vi "Measure vs B2Dv10.vi"() -> ()   [LabVIEW 2009]
doc: "This VI is an example operator panel.\n\nThe VI contains a table for the field values that may be configured manually, or loaded by checking the \"Prompt for File\" box. The data file should contain 3 columns of data, with each column delimited by a tab character.\n\nBefore the VI is executed, set the desired field units and coordinate system. Once the VI is started, follow the directions in the STATUS indicator to operate. Once a field value is achieved, it will be held indefinitely with no user intervention.\n\nThe present field is displayed in the selected units and coordinate system. The present field is queried once per second.\n\nIf a field point is specified that is outside the limits for the magnet, the VI will abort execution."
uses:
  <vilib>/Utility/file.llb/Read From Spreadsheet File (DBL).vi
panel:
  in  "AH":bool=TRUE
  in  "GPIB HP 2":string="13"
  in  "Wait between \nVectors":bool
  in  "Change\nPID\n(DetermineSIMPID.vi)":bool
  in  "Wait between \nVectors (ms)":u32=3000
  in  "X Axis":enum16{"B", "phi"}(ring)
  in  "Y Axis":T1(ring)=enum."HP (V)2"
  out "measured data":dbl[][](array[numeric])
  out "XY Graph":T2(graph)
  in  "Notes:":string="Datum: 16.01.12, Uhrzeit: 14:00, Sweep 0.15T/min,(measurevsB2Dv10.vi)), kapazitive Messung, leerer Sensor #1649_1, Referenzmessung, T=0.3K, Winkel 15° , optischer Probenstab, Gestell entfernt" caption="Notizen:"
  out "Messfile Refnum":refnum<file>
  in  "Measurement File":path=path "D:/UserData/Matthias/Messungen/#1649_leer/120116/120116_#1649_135deg_M1.txt"
  in  "Sample name:":string="#1649_1, leer"
  in  "HP 1":bool
  in  "GPIB HP":string="14"
  in  "HP 2":bool
  in  "LI 3":bool
  in  "GPIB L 3":string="8"
  in  "LI 2":bool
  in  "GPIB L 2":string="8"
  in  "LI 1":bool
  in  "GPIB L 1":string="8"
  out "Number of lines":i32=3
  in  "Operation":u16(ring)=1 items=["Stepwise", "Continous"]
  out "Ramp Rate along Vector (T/min)":dbl=0.2123426648592312 format="%.3f"
  out "Current Ramp Rate Z (T/min)":dbl=0.15014787650686168 format="%.3f"
  out "Current Ramp Rate Y (T/min)":dbl=0.15015 format="%.3f"
  in  "User defined Ramp Rate (T/min)":bool=TRUE
  in  "User defined Ramp Rate (T/min)":dbl=0.22 format="%.3f"
  in  "Z-Axis Communications Config":T3={"GPIB address"=22, "GPIB bus"=1, "connection ID"=refnum, "IP"="111.111.111.1", "Active Comm Interface"=0, "Serial Port"="", "Programmer Type"=0} {"Programmer Type" items=["Model 430", "Model 420"]; "Active Comm Interface" items=["TCP/IP (Model 430 Only)", "RS232", "IEEE488"]}
  in  "Max Ramp Rate - Y Axis (A/s)":dbl=0.055 format="%.3f"
  in  "Max Ramp Rate - Z Axis (A/s)":dbl=0.19 format="%.3f"
  in  "Magnitude Limit (kG)":dbl=45.1 format="%.3f"
  in  "Y-Axis Communications Config":T3={"GPIB address"=22, "GPIB bus"=1, "connection ID"=refnum, "IP"="111.111.111.2", "Active Comm Interface"=0, "Serial Port"="", "Programmer Type"=0} {"Programmer Type" items=["Model 430", "Model 420"]; "Active Comm Interface" items=["TCP/IP (Model 430 Only)", "RS232", "IEEE488"]}
  out "Cartesian Display (T)":T4={"Y-Axis Field (T)"=-1e-05, "Z-Axis Field (T)"=2.9999999999999997e-05} {"Z-Axis Field (T)" format="%.3f"; "Y-Axis Field (T)" format="%.3f"}
  in  "Starting index":i32=2
  in  "Normal color":u32(colorbox)=11711154
  in  "Highlight color":u32(colorbox)=16711680
  in  "Prompt for File?":bool
  out "Continue Execution?":bool=TRUE
  out "error out":T5
  in  "error in":T5
  out "STATUS":string="Zeroing vector."
  in  "Ramping Control":u16(ring)=4 items=["NEXT VECTOR", "RAMPING", "HOLDING", "PAUSE", "ZERO"]
  out "Cartesian Display (kG)":T6 {"Z-Axis Field (kG)" format="%.3f"; "Y-Axis Field (kG)" format="%.3f"}
  in  "Field Values":string[][](table)=[["4", "135"], ["-4", "135"], ["0", "0"]]
  out "Switch Heaters":bool=TRUE
  out "Polar Display (T)":T7={"q (degrees)"=315.0, "Field Magnitude (T)"=1.4142135623730951e-05} {"Field Magnitude (T)" format="%.3f"; "q (degrees)" format="%.3f"}
  out "Polar Display (kG)":T8 {"Field Magnitude (kG)" format="%.3f"; "q (degrees)" format="%.3f"}
  in  "Coordinate System":u16(ring)=1 items=["Cartesian", "Polar"]
  in  "Magnetic Field Units":u16(ring)=1 items=["kG", "Tesla"]
  # "kontinuirliche Messung mit PID off bei 0, geht nur im Cartesian mode!"
  # "Measurement Display"
  # "Measurement Settings"
  # "Magnet Settings"
  # "Max Ramp Rate z: 1.27 T/min\nMax Ramp Rate y: 0.17 T/min"
  # "Devices"
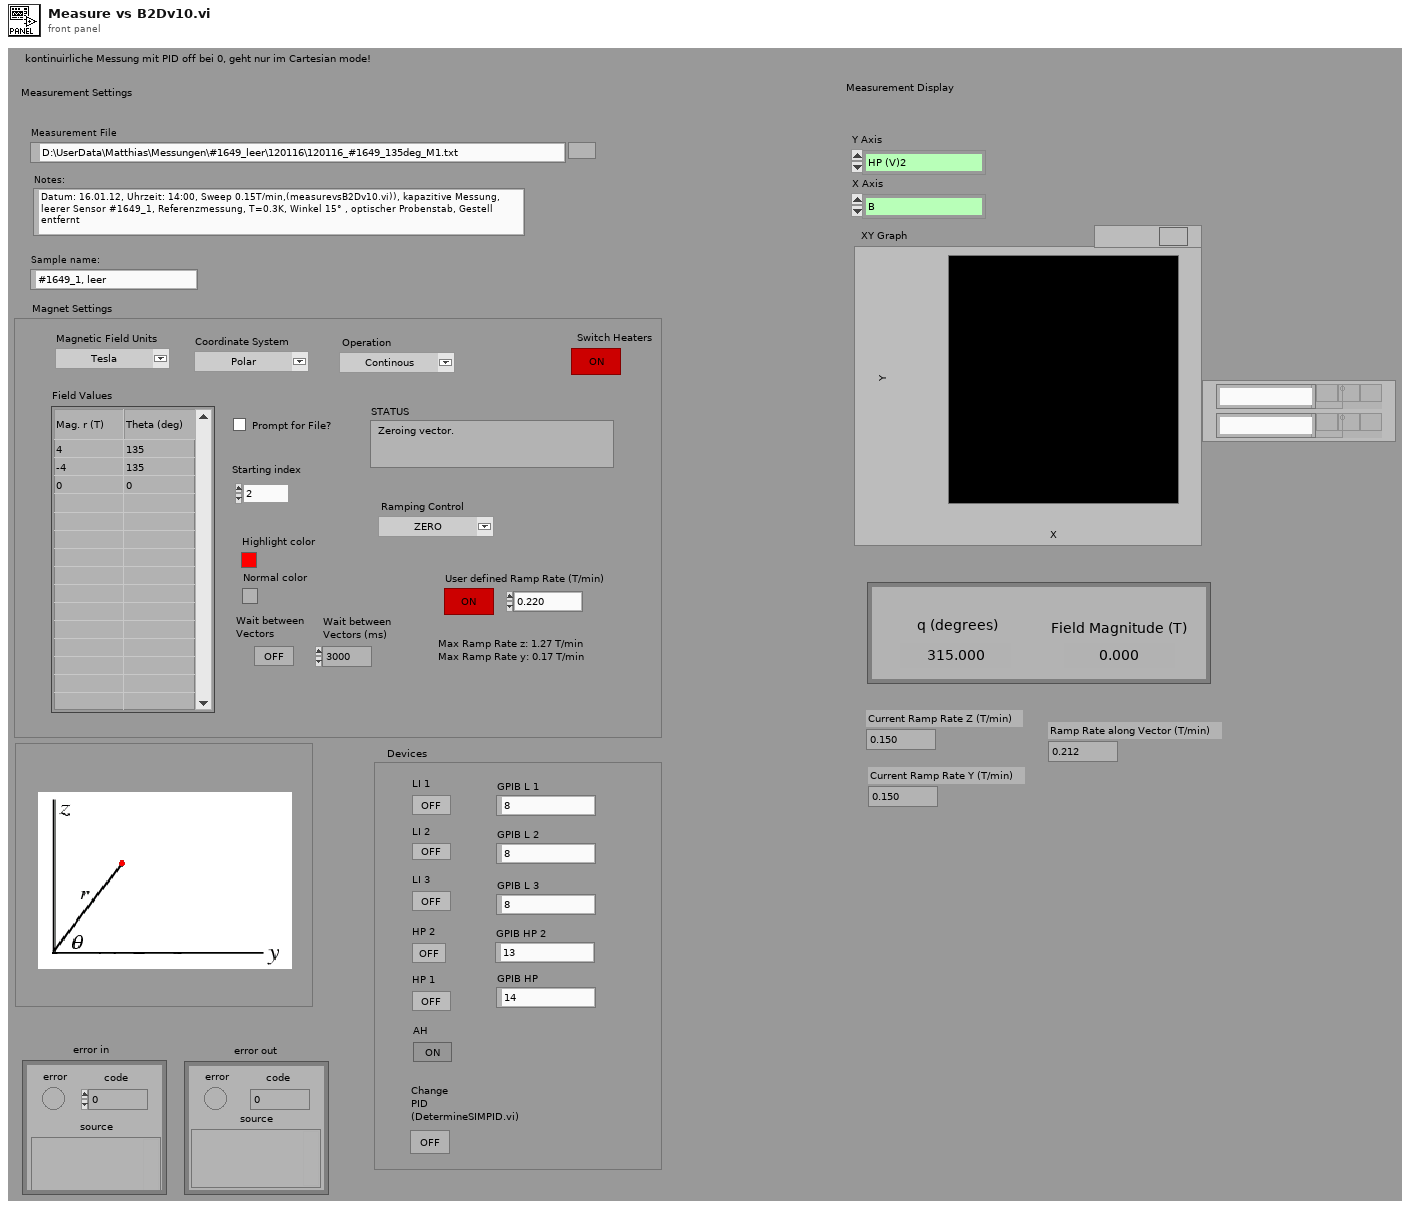
[diagram p1: front panel]
types:
  T1 = enum16{"B", "phi", "LI 1 Vx", "LI 1 phase", "LI 2 Vx", "LI 2 phase", "LI 3 Vx", "LI 3 phase", "LI 4 Vx", "LI 4 phase", "HP (V)", "HP (V)2", "AH C (pF)", "AH loss"}
  T2 = cluster{"measured data":dbl[], "measured data":dbl[]}
  T3 = cluster{"GPIB address":i16, "GPIB bus":i16, "connection ID":refnum<k5>, "IP":string, "Active Comm Interface":u16, "Serial Port":refnum<visa-resource-name>, "Programmer Type":u16}
  T4 = cluster{"Y-Axis Field (T)":dbl, "Z-Axis Field (T)":dbl}
  T5 = cluster{"error":bool, "code":i32, "source":string}
  T6 = cluster{"Y-Axis Field (kG)":dbl, "Z-Axis Field (kG)":dbl}
  T7 = cluster{"q (degrees)":dbl, "Field Magnitude (T)":dbl}
  T8 = cluster{"q (degrees)":dbl, "Field Magnitude (kG)":dbl}
  T9 = enum16{"", "RAMPING", "HOLDING", "PAUSED", "MANUAL UP", "MANUAL DOWN", "ZEROING CURRENT", "QUENCH DETECTED", "HEATING SWITCH"}
  T10 = enum16{"", "RAMPING", "HOLDING", "PAUSED", "MANUAL UP", "MANUAL DOWN", "ZEROING CURRENT", "QUENCH DETECTED", "HEATING SWITCH", "AT ZER0", "COOLING SWITCH"}
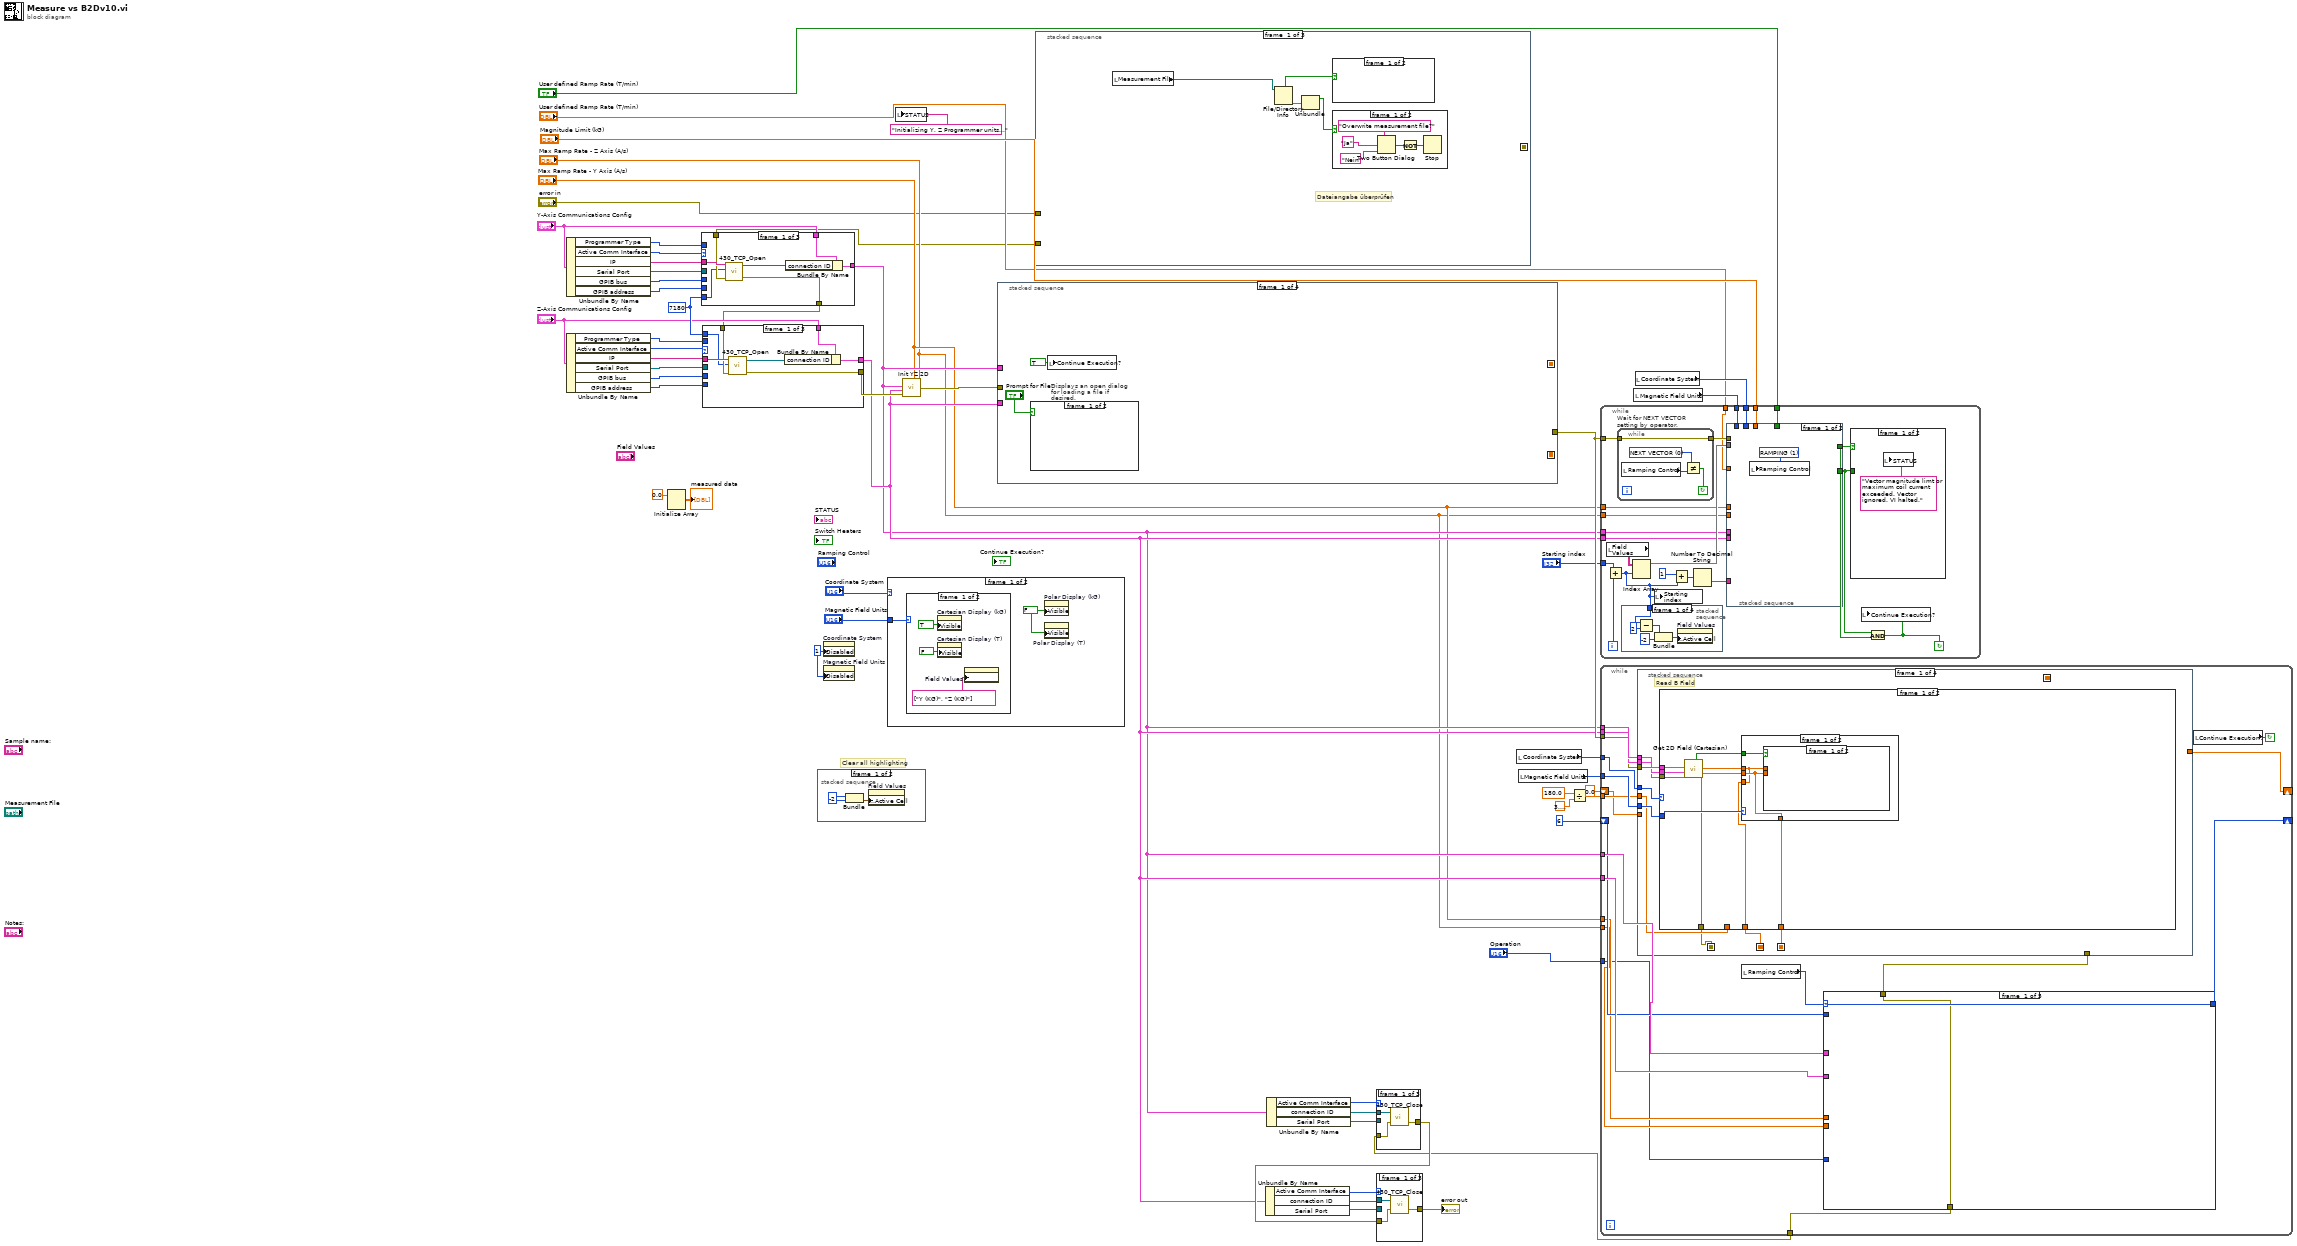
[diagram p0: block diagram]
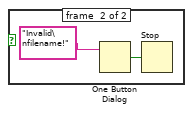
[diagram p3: hidden frame]
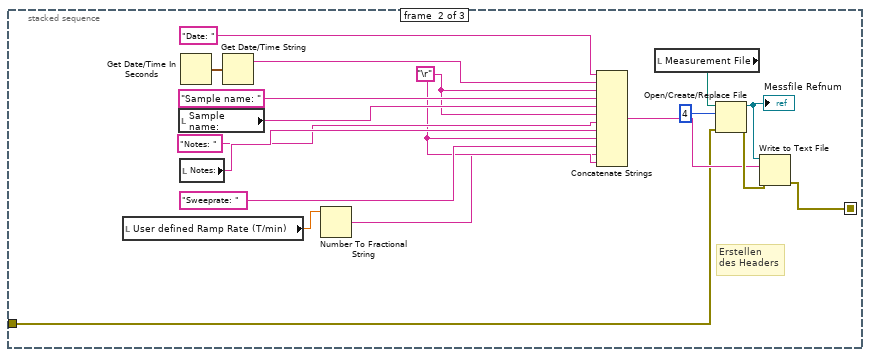
[diagram p4: hidden frame]
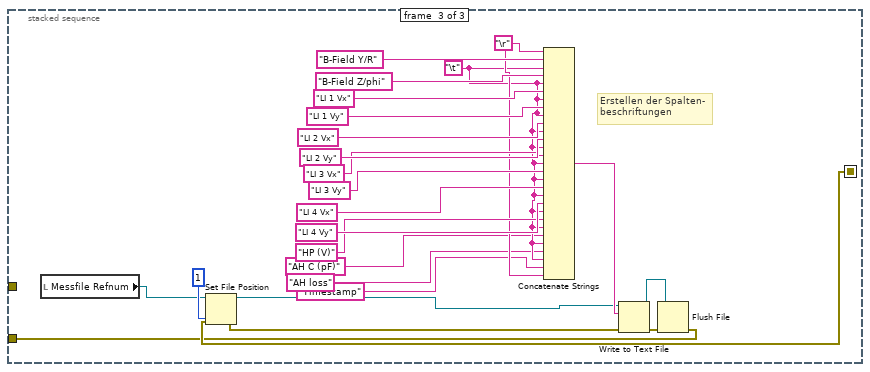
[diagram p5: hidden frame]
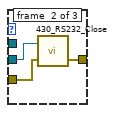
[diagram p6: hidden frame]
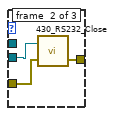
[diagram p8: hidden frame]
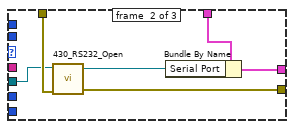
[diagram p10: hidden frame]
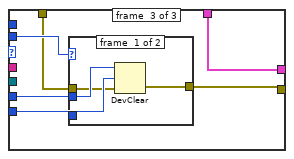
[diagram p11: hidden frame]
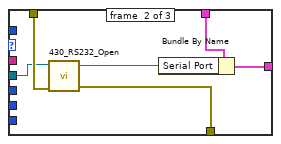
[diagram p13: hidden frame]
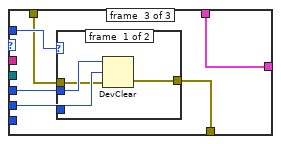
[diagram p14: hidden frame]
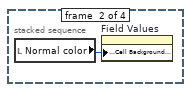
[diagram p16: hidden frame]
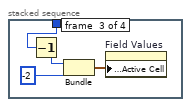
[diagram p17: hidden frame]
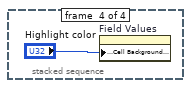
[diagram p18: hidden frame]
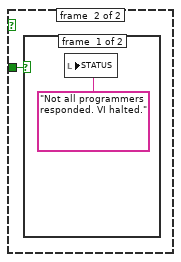
[diagram p19: hidden frame]
diagram:
  w39 = 7180 ("TCP Port")
  w52 = u8 1 ("Write Attribute")
  # "Clear all highlighting"
  n1 = Unbundle By Name("Z-Axis Communications Config") -> ("Programmer Type"=w15:u16, "Active Comm Interface"=w38:u16, "IP"=w35:string, "Serial Port"=w34:refnum<visa-resource-name>, "GPIB bus"=w14:i16, "GPIB address"=w13:i16)
  n2 = Unbundle By Name("Y-Axis Communications Config") -> ("Programmer Type"=w9:u16, "Active Comm Interface"=w37:u16, "IP"=w36:string, "Serial Port"=w33:refnum<visa-resource-name>, "GPIB bus"=w10:i16, "GPIB address"=w11:i16)
  n3 = Initialize Array(0.0 ("element")) -> (→"measured data":dbl[][])  [unwired: 2 in]
  n4 = stacked-sequence {
    frame #0 {
      w55 = -2
      n5 = Bundle(w55, w55) -> (w56:cluster{i32, i32})  [unwired: 1 in]
      n6 = property on="Field Values" class="Tbl (strict)"("Active Cell:Active Cell"=w56) -> ()  [unwired: 2 in, 2 out]
    }
    frame #1 {
      n7 = property on="Field Values" class="Tbl (strict)"("Active Cell:Cell Background Color"="Normal color") -> ()  [unwired: 2 in, 2 out]
    }
  }
  n8 = property on="Coordinate System" class="Ring (strict)"("Disabled"=w52) -> ()  [unwired: 2 in, 2 out]
  n9 = property on="Magnetic Field Units" class="Ring (strict)"("Disabled"=w52) -> ()  [unwired: 2 in, 2 out]
  n10 = case shown="0, Default" "Coordinate System" {
    tunnel: "Magnetic Field Units" -> [w59 w67]
    frame #0 {
      w58 = FALSE ("Write Attribute")
      (unwired) FALSE ("Write Attribute")
      (unwired) TRUE ("Write Attribute")
      n11 = case shown="1" w59 {
        frame #0 {
          n12 = property on="Cartesian Display (kG)" class="Cluster (strict)"("Visible"=TRUE ("Write Attribute")) -> ()  [unwired: 2 in, 2 out]
          n13 = property on="Cartesian Display (T)" class="Cluster (strict)"("Visible"=FALSE ("Write Attribute")) -> ()  [unwired: 2 in, 2 out]
          n14 = property on="Field Values" class="Tbl (strict)"("Column Header Strings[]"=string[] ["Y (KG)", "Z (KG)"] ("Write Attribute")) -> ()  [unwired: 2 in, 2 out]
        }
        frame #1 {
          n15 = property on="Cartesian Display (kG)" class="Cluster (strict)"("Visible"=FALSE ("Write Attribute")) -> ()  [unwired: 2 in, 2 out]
          n16 = property on="Cartesian Display (T)" class="Cluster (strict)"("Visible"=TRUE ("Write Attribute")) -> ()  [unwired: 2 in, 2 out]
          n17 = property on="Field Values" class="Tbl (strict)"("Column Header Strings[]"=string[] ["Y (T)", "Z (T)"] ("Write Attribute")) -> ()  [unwired: 2 in, 2 out]
        }
      }
      n18 = property on="Polar Display (kG)" class="Clust (strict)"("Visible"=w58) -> ()  [unwired: 2 in, 2 out]
      n19 = property on="Polar Display (T)" class="Clust (strict)"("Visible"=w58) -> ()  [unwired: 2 in, 2 out]
    }
    frame #1 {
      (unwired) FALSE ("Write Attribute")
      (unwired) TRUE ("Write Attribute")
      w66 = FALSE ("Write Attribute")
      n20 = case shown="1" w67 {
        frame #0 {
          n21 = property on="Polar Display (kG)" class="Clust (strict)"("Visible"=TRUE ("Write Attribute")) -> ()  [unwired: 2 in, 2 out]
          n22 = property on="Polar Display (T)" class="Clust (strict)"("Visible"=FALSE ("Write Attribute")) -> ()  [unwired: 2 in, 2 out]
          n23 = property on="Field Values" class="Tbl (strict)"("Column Header Strings[]"=string[] ["Mag. r (KG)", "Theta (deg)"] ("Write Attribute")) -> ()  [unwired: 2 in, 2 out]
        }
        frame #1 {
          n24 = property on="Polar Display (kG)" class="Clust (strict)"("Visible"=FALSE ("Write Attribute")) -> ()  [unwired: 2 in, 2 out]
          n25 = property on="Polar Display (T)" class="Clust (strict)"("Visible"=TRUE ("Write Attribute")) -> ()  [unwired: 2 in, 2 out]
          n26 = property on="Field Values" class="Tbl (strict)"("Column Header Strings[]"=string[] ["Mag. r (T)", "Theta (deg)"] ("Write Attribute")) -> ()  [unwired: 2 in, 2 out]
        }
      }
      n27 = property on="Cartesian Display (kG)" class="Cluster (strict)"("Visible"=w66) -> ()  [unwired: 2 in, 2 out]
      n28 = property on="Cartesian Display (T)" class="Cluster (strict)"("Visible"=w66) -> ()  [unwired: 2 in, 2 out]
    }
  }
  n29 = local write "STATUS"("Initializing Y, Z Programmer units..." ("STATUS")) -> ()
  n30 = stacked-sequence {
    seq-local: [_ w85 _] -> [_ _ w109]
    tunnel: "error in" -> [_ w86 _]
    tunnel: [_ _ w108] -> w4
    frame #0 {
      # "Dateiangabe überprüfen"
      n31 = local read "Measurement File"() -> (w77:path)
      n32 = File/Directory Info(path=w77) -> (directory=w75:bool, error out=w76:errorcluster)  [unwired: 1 in, 5 out]
      n33 = Unbundle(w76) -> ("status"=w74:bool)  [unwired: 2 out]
      n34 = case shown="False" w75 {
        frame #0 {
        }
        frame #1 {
          n35 = One Button Dialog(message="Invalid\nfilename!") -> (true=w83:bool)  [unwired: 1 in]
          n36 = Stop(stop? (T)=w83) -> ()
        }
      }
      n37 = case shown="False" w74 {
        frame #0 {
          n38 = Two Button Dialog(message="Overwrite measurement file?", 1:"Nein", 2:"Ja") -> (T button?=w79:bool)
          n39 = Not(x=w79) -> (.not. x?=w78:bool)
          n40 = Stop(stop? (T)=w78) -> ()
        }
        frame #1 {
        }
      }
    }
    frame #1 {
      w89 = "\r"
      # "Erstellen\ndes Headers"
      n41 = local read "User defined Ramp Rate (T/min)"() -> (w88:dbl)
      n42 = local read "Sample name:"() -> (w95:string)
      n43 = local read "Notes:"() -> (w97:string)
      n44 = Get Date/Time In Seconds() -> (seconds since 1Jan1904=w91:timestamp)
      n45 = Get Date/Time String(seconds (now)=w91) -> (date string=w93:string)  [unwired: 2 in, 1 out]
      n46 = Number To Fractional String(number=w88) -> (F-format string=w87:string)  [unwired: 3 in]
      n47 = Concatenate Strings("Date: ", w93, w89, "Sample name: ", w95, w89, "Notes: ", w97, w89, "Sweeprate: ", w87, w89) -> (w101:string)
      n48 = local read "Measurement File"() -> (w98:path)
      n49 = Open/Create/Replace File(file path (use dialog)=w98, error in=w86, operation (0:open)=4) -> (refnum out=w100:refnum<file>, error out=w102:errorcluster)  [unwired: 3 in, 1 out]
      "Messfile Refnum" <- w100
      n50 = Write to Text File(file (use dialog)=w100, text=w101, error in=w102) -> (error out=w85:errorcluster)  [unwired: 1 in, 2 out]
    }
    frame #2 {
      w105 = "\t"
      w107 = "\r"
      # "Erstellen der Spalten-\nbeschriftungen"
      n51 = local read "Messfile Refnum"() -> (w116:refnum<file>)
      n52 = Set File Position(refnum=w116, from (0:start)=1, error in=w109) -> (refnum out=w122:refnum<file>, error out=w124:errorcluster)  [unwired: 1 in]
      n53 = Concatenate Strings(w107, "B-Field Y/R", w105, "B-Field Z/phi", w105, "LI 1 Vx", w105, "LI 1 Vy", w105, "LI 2 Vx", w105, "LI 2 Vy", w105, "LI 3 Vx", w105, "LI 3 Vy", w105, "LI 4 Vx", w105, "LI 4 Vy", w105, "HP (V)", w105, "AH C (pF)" ("string"), w105, "AH loss" ("string"), w105, "Timestamp", w107) -> (w123:string)
      n54 = Write to Text File(file (use dialog)=w122, text=w123, error in=w124) -> (refnum out=w126:refnum<file>, error out=w125:errorcluster)  [unwired: 1 in, 1 out]
      n55 = Flush File(refnum=w126, error in=w125) -> (error out=w108:errorcluster)  [unwired: 1 out]
    }
  }
  n56 = case shown="0, Default" w37 {
    tunnel: w36 -> [w134 _ _]
    tunnel: w4 -> [w133 w140 w142]
    tunnel: "Y-Axis Communications Config" -> [w132 w135 w146]
    tunnel: [w130 w138 w146] -> w22
    tunnel: [w129 w139 w141] -> w12
    tunnel: w39 -> [w128 _ _]
    tunnel: w33 -> [_ w136 _]
    tunnel: w11 -> [_ _ w145]
    tunnel: w10 -> [_ _ w144]
    tunnel: w9 -> [_ _ w143]
    frame #0 {
      n57 = call <userlib>:"430_TCP_Open.vi"("IP Address"=w134, "TCP Port"=w128, "error in (no error)"=w133) -> ("connection ID"=w131:refnum<k5>, "error out"=w129:errorcluster)  [unwired: 3 in, 1 out]
      n58 = Bundle By Name(cluster=w132, "connection ID"=w131) -> (w130:T3)
    }
    frame #1 {
      n59 = call <userlib>:"430_RS232_Open.vi"("VISA resource name"=w136, "error in (no error)"=w140) -> ("VISA resource name out"=w137:refnum<visa-resource-name>, "error out"=w139:errorcluster)  [unwired: 5 in]
      n60 = Bundle By Name(cluster=w135, "Serial Port"=w137) -> (w138:T3)
    }
    frame #2 {
      n61 = case shown="1" w143 {
        tunnel: w144 -> [w150 _]
        tunnel: w145 -> [w149 _]
        tunnel: w142 -> [w148 w151]
        tunnel: [w147 w151] -> w141
        frame #0 {
          n62 = DevClear(2:w148, 3:w149, 4:w150) -> (0:w147:errorcluster)  [unwired: 1 out]
        }
        frame #1 {
        }
      }
    }
  }
  n63 = case shown="0, Default" w38 {
    tunnel: w35 -> [w158 _ _]
    tunnel: w12 -> [w157 w164 w166]
    tunnel: [w156 w163 w165] -> w32
    tunnel: "Z-Axis Communications Config" -> [w155 w161 w170]
    tunnel: [w153 w162 w170] -> w23
    tunnel: w39 -> [w152 _ _]
    tunnel: w34 -> [_ w159 _]
    tunnel: w15 -> [_ _ w169]
    tunnel: w14 -> [_ _ w168]
    tunnel: w13 -> [_ _ w167]
    frame #0 {
      n64 = call <userlib>:"430_TCP_Open.vi"("IP Address"=w158, "TCP Port"=w152, "error in (no error)"=w157) -> ("connection ID"=w154:refnum<k5>, "error out"=w156:errorcluster)  [unwired: 3 in, 1 out]
      n65 = Bundle By Name(cluster=w155, "connection ID"=w154) -> (w153:T3)
    }
    frame #1 {
      n66 = call <userlib>:"430_RS232_Open.vi"("VISA resource name"=w159, "error in (no error)"=w164) -> ("VISA resource name out"=w160:refnum<visa-resource-name>, "error out"=w163:errorcluster)  [unwired: 5 in]
      n67 = Bundle By Name(cluster=w161, "Serial Port"=w160) -> (w162:T3)
    }
    frame #2 {
      n68 = case shown="0, Default" w169 {
        tunnel: w168 -> [w174 _]
        tunnel: w167 -> [w173 _]
        tunnel: w166 -> [w172 w175]
        tunnel: [w171 w175] -> w165
        frame #0 {
          n69 = DevClear(2:w172, 3:w173, 4:w174) -> (0:w171:errorcluster)  [unwired: 1 out]
        }
        frame #1 {
        }
      }
    }
  }
  n70 = call <userlib>:"Init YZ 2D.vi"("Max Ramp Rate Z-axis"="Max Ramp Rate - Z Axis (A/s)", "Max Ramp Rate Y-axis"="Max Ramp Rate - Y Axis (A/s)", "error in"=w32, "Z-Axis Communications Config"=w23, "Y-Axis Communications Config"=w22) -> ("error out"=w50:T5)  [unwired: 5 in]
  n71 = stacked-sequence {
    seq-local: [_ w183 _ _] -> [_ _ w230 _]
    seq-local: [_ w182 _ _] -> [_ _ w229 _]
    tunnel: w23 -> [_ w185 _ _]
    tunnel: w50 -> [_ w186 _ _]
    tunnel: [_ w181 _ _] -> w46
    tunnel: w22 -> [_ w184 _ _]
    frame #0 {
      n72 = case "Displays an open dialog for loading a file if desired." shown="True" "Prompt for File?" {
        frame #0 {
        }
        frame #1 {
          n73 = call-poly <vilib>:"Read From Spreadsheet File.vi"() -> ("all rows"=w180:dbl[][])  [unwired: 7 in, 4 out]
          n74 = Number To Fractional String(number=w180, precision (6)=i16 4) -> (F-format string=w179:string[][])  [unwired: 2 in]
          n75 = local write "Field Values"(w179) -> ()
        }
      }
      n76 = local write "Continue Execution?"(TRUE ("Continue Execution?")) -> ()
    }
    frame #1 {
      w194 = u16 3 items=["NEXT VECTOR", "RAMPING", "HOLDING", "PAUSE", "ZERO"] ("Ramping Control")
      n77 = call <userlib>:"Get Switch Present.vi"("error in"=w186, "Communications Config"=w184) -> ("error out"=w190:T5, "Switch Present?"=w191:bool)
      n78 = case shown="True" w191 {
        tunnel: w190 -> [w212 w221]
        tunnel: w184 -> [_ w214]
        tunnel: [0.0 w218] -> w182
        tunnel: [w212 w220] -> w189
        frame #0 {
        }
        frame #1 {
          n79 = call <userlib>:"Get Switch Heater Time.vi"("error in"=w221, "Communications Config"=w214) -> ("error out"=w217:T5, "Switch Heating Time (secs)"=w219:dbl)
          n80 = call <userlib>:"Get Switch Heater.vi"("error in"=w217, "Communications Config"=w214) -> ("error out"=w216:T5, "Switch Heater Indicator"=w215:bool)
          n81 = case shown="False" w215 {
            tunnel: [w226 w227] -> w220
            tunnel: w219 -> [w224 _]
            tunnel: [w224 0.0] -> w218
            tunnel: w216 -> [w222 w227]
            tunnel: w214 -> [w223 _]
            frame #0 {
              n82 = call <userlib>:"Set Switch Heater.vi"("error in"=w222, "Switch Heater Control"=TRUE, "Communications Config"=w223) -> ("error out"=w226:T5)
            }
            frame #1 {
            }
          }
        }
      }
      n83 = call <userlib>:"Get Switch Present.vi"("error in"=w189, "Communications Config"=w185) -> ("error out"=w187:T5, "Switch Present?"=w188:bool)
      n84 = case shown="True" w188 {
        tunnel: w187 -> [w195 w204]
        tunnel: w185 -> [_ w197]
        tunnel: [0.0 w201] -> w183
        tunnel: [w195 w203] -> w181
        frame #0 {
        }
        frame #1 {
          n85 = call <userlib>:"Get Switch Heater Time.vi"("error in"=w204, "Communications Config"=w197) -> ("error out"=w200:T5, "Switch Heating Time (secs)"=w202:dbl)
          n86 = call <userlib>:"Get Switch Heater.vi"("error in"=w200, "Communications Config"=w197) -> ("error out"=w199:T5, "Switch Heater Indicator"=w198:bool)
          n87 = case shown="False" w198 {
            tunnel: [w205 w210] -> w203
            tunnel: w202 -> [w208 _]
            tunnel: [w208 0.0] -> w201
            tunnel: w199 -> [w206 w210]
            tunnel: w197 -> [w207 _]
            frame #0 {
              n88 = call <userlib>:"Set Switch Heater.vi"("error in"=w206, "Switch Heater Control"=TRUE, "Communications Config"=w207) -> ("error out"=w205:T5)
            }
            frame #1 {
            }
          }
        }
      }
      n89 = local write "Ramping Control"(w194) -> ()
      n90 = local write "Switch Heaters"(TRUE ("Switch Heater Control")) -> ()
      n91 = property on="Switch Heaters" class="Boolean (strict)"("Disabled"=u8 1 ("Write Attribute")) -> ()  [unwired: 2 in, 2 out]
    }
    frame #2 {
      n92 = Max & Min(x=w230, y=w229) -> (max(x,y)=w231:dbl)  [unwired: 1 out]
      n93 = local write "STATUS"("Heating switches..." ("STATUS")) -> ()
      n94 = Add(x=w231, y=2) -> (x+y=w235:dbl)
      n95 = property on="Ramping Control" class="Ring (strict)"("Disabled"=u8 1 ("Write Attribute")) -> ()  [unwired: 2 in, 2 out]
      n96 = Multiply(x=w235, y=1000) -> (x*y=w234:dbl)
      n97 = Wait (ms)(milliseconds to wait=w234) -> ()  [unwired: 1 out]
    }
    frame #3 {
      n98 = property on="Ramping Control" class="Ring (strict)"("Disabled"=u8 0 ("Write Attribute")) -> ()  [unwired: 2 in, 2 out]
      n99 = local write "STATUS"("Ready to ramp to first vector. Set Ramping Mode to NEXT VECTOR to begin." ("STATUS")) -> ()
      n100 = local read "Field Values"() -> (w240:string[][])
      n101 = Array Size(array=w240) -> (size(s)=w239:i32[])
      n102 = Index Array(array=w239, index=0) -> (element=→"Number of lines":i32)
    }
  }
  n103 = Unbundle By Name(w23) -> ("Active Comm Interface"=w29:u16, "connection ID"=w28:refnum<k5>, "Serial Port"=w27:refnum<visa-resource-name>)
  n104 = Unbundle By Name(w22) -> ("Active Comm Interface"=w30:u16, "connection ID"=w26:refnum<k5>, "Serial Port"=w25:refnum<visa-resource-name>)
  n105 = local read "Coordinate System"() -> (w47:u16)
  n106 = local read "Magnetic Field Units"() -> (w45:u16)
  n107 = Divide(x=180.0, y=3.141592653589793) -> (x/y=w42:dbl)
  n108 = while {
    shift-left: u16 6 ("Ramping Control") -> [w250]
    shift-right: [w251] -> _
    tunnel: [w253] -> w24
    tunnel: w23 -> [w254]
    tunnel: w22 -> [w255]
    tunnel: w42 -> [w257]
    tunnel: w45 -> [w258]
    tunnel: w46 -> [w259]
    tunnel: w23 -> [w260]
    tunnel: w22 -> [w261]
    tunnel: w47 -> [w262]
    tunnel: "Max Ramp Rate - Y Axis (A/s)" -> [w249]
    tunnel: "Max Ramp Rate - Z Axis (A/s)" -> [w248]
    tunnel: "Operation" -> [w247]
    shift-right: [w245] -> _
    shift-left: 0.0 -> [w244]
    stop <- w252 continue-if-true
    n109 = stacked-sequence {
      seq-local: [w265 _ _ _] -> [_ _ w389 _]
      seq-local: [w264 _ _ _] -> [_ w338 w386 _]
      seq-local: [w263 _ _ _] -> [_ w339 w387 _]
      seq-local: [_ _ w374 _] -> [_ _ _ w459]
      tunnel: w262 -> [w271 _ _ w457]
      tunnel: w261 -> [w270 _ _ _]
      tunnel: w260 -> [w269 _ _ _]
      tunnel: w259 -> [w268 _ _ _]
      tunnel: w258 -> [w267 _ _ _]
      tunnel: w257 -> [w266 _ _ _]
      tunnel: [_ _ w388 _] -> w246
      tunnel: [_ w341 _ _] -> w245
      tunnel: w244 -> [_ w340 _ _]
      frame #0 {
        # "Read B Field"
        n110 = case shown="0, Default" w271 {
          tunnel: w270 -> [w281 w304]
          tunnel: w269 -> [w280 w303]
          tunnel: w268 -> [w279 w302]
          tunnel: w267 -> [w278 w301]
          tunnel: w266 -> [_ w300]
          tunnel: [w274 w299] -> w265
          tunnel: [w273 w297] -> w264
          tunnel: [w272 w298] -> w263
          frame #0 {
            n111 = call <userlib>:"Get 2D Field (Cartesian).vi"("Y-Axis Communications Config"=w281, "Z-Axis Communications Config"=w280, "error in"=w279) -> ("All Instruments Responded?"=w275:bool, "Y-Axis Field (kG)"=w277:dbl, "Z-Axis Field (kG)"=w276:dbl, "error out"=w274:T5)  [unwired: 2 in]
            n112 = case shown="0, Default" w278 {
              tunnel: w277 -> [w282 w290]
              tunnel: w276 -> [w283 w291]
              tunnel: w275 -> [w284 w293]
              tunnel: [w283 w289] -> w273
              tunnel: [w282 w288] -> w272
              frame #0 {
                n113 = case shown="True" w284 {
                  tunnel: w282 -> [_ w286]
                  tunnel: w283 -> [_ w285]
                  frame #0 {
                  }
                  frame #1 {
                    n114 = Bundle("Y-Axis Field (kG)"=w286, "Z-Axis Field (kG)"=w285) -> (→"Cartesian Display (kG)":T6)  [unwired: 1 in]
                  }
                }
              }
              frame #1 {
                w292 = 0.1 ("y")
                n115 = Multiply(x=w290, y=w292) -> (x*y=w288:dbl)
                n116 = Multiply(x=w291, y=w292) -> (x*y=w289:dbl)
                n117 = case shown="True" w293 {
                  tunnel: w288 -> [_ w296]
                  tunnel: w289 -> [_ w295]
                  frame #0 {
                  }
                  frame #1 {
                    n118 = Bundle(w296, w295) -> (→"Cartesian Display (T)":cluster{dbl, dbl})  [unwired: 1 in]
                  }
                }
              }
            }
          }
          frame #1 {
            n119 = stacked-sequence {
              tunnel: w304 -> [w315]
              tunnel: w303 -> [w314]
              tunnel: w302 -> [w313]
              tunnel: w301 -> [w312]
              tunnel: w300 -> [w309]
              tunnel: [w307] -> w299
              tunnel: [w306] -> w297
              tunnel: [w305] -> w298
              frame #0 {
                # "Field"
                n120 = call <userlib>:"Get 2D Field (Polar).vi"("Y-Axis Communications Config"=w315, "Z-Axis Communications Config"=w314, "error in"=w313) -> ("All Instruments Responded?"=w308:bool, "Radial (r) Field (kG)"=w311:dbl, "q (radians)"=w310:dbl, "error out"=w307:T5)  [unwired: 2 in]
                n121 = case shown="1" w312 {
                  tunnel: w311 -> [w317 w329]
                  tunnel: w310 -> [w319 w328]
                  tunnel: w309 -> [w318 w327]
                  tunnel: w308 -> [w320 w326]
                  tunnel: [w317 w324] -> w306
                  tunnel: [w316 w325] -> w305
                  frame #0 {
                    n122 = Multiply(x=w319, y=w318) -> (x*y=w316:dbl)
                    n123 = case shown="True" w320 {
                      tunnel: w317 -> [_ w321]
                      tunnel: w316 -> [_ w322]
                      frame #0 {
                      }
                      frame #1 {
                        n124 = Bundle(w322, "Radial (r) Field (kG)"=w321) -> (→"Polar Display (kG)":cluster{dbl, "Radial (r) Field (kG)":dbl})  [unwired: 1 in]
                      }
                    }
                  }
                  frame #1 {
                    n125 = Multiply(x=w329, y=0.1) -> (x*y=w325:dbl)
                    n126 = Multiply(x=w328, y=w327) -> (x*y=w324:dbl)
                    n127 = case shown="True" w326 {
                      tunnel: w325 -> [_ w331]
                      tunnel: w324 -> [_ w332]
                      frame #0 {
                      }
                      frame #1 {
                        n128 = Bundle(w332, w331) -> (→"Polar Display (T)":cluster{dbl, dbl})  [unwired: 1 in]
                      }
                    }
                  }
                }
              }
            }
          }
        }
      }
      frame #1 {
        # "Change PID"
        n129 = Square(x=w339) -> (x^2=w336:dbl)
        n130 = Square(x=w338) -> (x^2=w337:dbl)
        n131 = Add(x=w336, y=w337) -> (x+y=w335:dbl)
        n132 = Square Root(x=w335) -> (sqrt(x)=w334:dbl)
        n133 = case shown="True" "Change\nPID\n(DetermineSIMPID.vi)" {
          tunnel: w334 -> [_ w353]
          tunnel: [_ w349] -> w341
          tunnel: w340 -> [_ w351]
          frame #0 {
          }
          frame #1 {
            n134 = Absolute Value(x=w353) -> (abs(x)=w349:dbl)
            n135 = Less Or Equal?(x=w349, y=0.07 ("upper limit")) -> (x <= y?=w346:bool)
            n136 = Greater?(x=w351, y=0.07 ("upper limit")) -> (0:w347:bool)
            n137 = Not(x=w347) -> (.not. x?=w344:bool)
            n138 = Not(x=w346) -> (.not. x?=w345:bool)
            n139 = And(x=w347, y=w346) -> (x .and. y?=w352:bool)
            n140 = And(x=w344, y=w345) -> (x .and. y?=w343:bool)
            n141 = case shown="True" w352 {
              frame #0 {
              }
              frame #1 {
                n142 = stacked-sequence {
                  frame #0 {
                    n143 = call "SIM960Poff.vi"("off/on (0/1)"="0", "Port Num- PID"="1", "GPIB-Adress"="2") -> ()  [unwired: 9 in]
                  }
                  frame #1 {
                    n144 = call "SIM960Poff.vi"("off/on (0/1)"="0", "Port Num- PID"="3", "GPIB-Adress"="2") -> ()  [unwired: 9 in]
                  }
                  frame #2 {
                    n145 = call "SIM960ChangeSignP.vi"("Port Num- PID"="1", "GPIB-Adress"="2") -> ()  [unwired: 10 in]
                  }
                }
              }
            }
            n146 = case shown="True" w343 {
              frame #0 {
              }
              frame #1 {
                n147 = stacked-sequence {
                  frame #0 {
                    n148 = call "SIM960Poff.vi"("off/on (0/1)"="1", "Port Num- PID"="3", "GPIB-Adress"="2") -> ()  [unwired: 9 in]
                  }
                  frame #1 {
                    n149 = call "SIM960Poff.vi"("off/on (0/1)"="1", "Port Num- PID"="1", "GPIB-Adress"="2") -> ()  [unwired: 9 in]
                  }
                }
              }
            }
          }
        }
      }
      frame #2 {
        w373 = u16 2 items=["NEXT VECTOR", "RAMPING", "HOLDING", "PAUSE", "ZERO"] ("Ramping Control")
        # "Zeile in Datei schreiben"
        # "Read and Save Devices"
        n150 = stacked-sequence {
          tunnel: [w401 _ _ _ _ _ _] -> w385
          tunnel: [w400 _ _ _ _ _ _] -> w384
          tunnel: [_ w414 _ _ _ _ _] -> w381
          tunnel: [_ w412 _ _ _ _ _] -> w380
          tunnel: [_ _ w424 _ _ _ _] -> w379
          tunnel: [_ _ w423 _ _ _ _] -> w378
          tunnel: [_ _ _ w435 _ _ _] -> w377
          tunnel: [_ _ _ 0.0 _ _ _] -> w376
          tunnel: [_ _ _ _ w441 _ _] -> w375
          tunnel: [_ _ _ _ _ _ w453] -> w370
          tunnel: [_ _ _ _ _ w448 _] -> w369
          tunnel: [_ _ _ _ _ w447 _] -> w368
          frame #0 {
            n151 = case shown="True" "LI 1" {
              tunnel: ["0" ("Antwort2") w408] -> w403
              tunnel: ["0" ("Antwort1") w407] -> w402
              frame #0 {
              }
              frame #1 {
                n152 = call "LI-Ansteuerung.vi"("Frage2"="OUTP? 4", "Frage1"="OUTP? 1", "address string"="GPIB L 1") -> ("Antwort2"=w408:string, "Antwort1"=w407:string)
              }
            }
            n153 = Fract/Exp String To Number(string=w403) -> (number=w400:dbl)  [unwired: 3 in, 1 out]
            n154 = Fract/Exp String To Number(string=w402) -> (number=w401:dbl)  [unwired: 3 in, 1 out]
          }
          frame #1 {
            n155 = case shown="False" "LI 2" {
              tunnel: [w417 w419] -> w413
              tunnel: [w417 w418] -> w415
              frame #0 {
                w417 = "0" ("Antwort1")
              }
              frame #1 {
                n156 = call "LI-Ansteuerung.vi"("Frage2"="OUTP? 4", "Frage1"="OUTP? 1", "address string"="GPIB L 2") -> ("Antwort2"=w419:string, "Antwort1"=w418:string)
              }
            }
            n157 = Fract/Exp String To Number(string=w413) -> (number=w412:dbl)  [unwired: 3 in, 1 out]
            n158 = Fract/Exp String To Number(string=w415) -> (number=w414:dbl)  [unwired: 3 in, 1 out]
          }
          frame #2 {
            n159 = case shown="False" "LI 3" {
              tunnel: [w428 w430] -> w425
              tunnel: [w428 w429] -> w426
              frame #0 {
                w428 = "0" ("Antwort1")
              }
              frame #1 {
                n160 = call "LI-Ansteuerung.vi"("Frage2"="OUTP? 4", "Frage1"="OUTP? 1", "address string"="GPIB L 3") -> ("Antwort2"=w430:string, "Antwort1"=w429:string)
              }
            }
            n161 = Fract/Exp String To Number(string=w426) -> (number=w424:dbl)  [unwired: 3 in, 1 out]
            n162 = Fract/Exp String To Number(string=w425) -> (number=w423:dbl)  [unwired: 3 in, 1 out]
          }
          frame #3 {
            n163 = case shown="False" "HP 2" {
              tunnel: [0.0 ("Voltage") w438] -> w435
              frame #0 {
              }
              frame #1 {
                n164 = call "HP-ReadVoltagev2.vi"("String"="meas:volt:dc? 10,0.001", "HP-Mulitmeter\nGPIB Address"="GPIB HP 2") -> ("Voltage"=w438:dbl)  [unwired: 9 in]
              }
            }
          }
          frame #4 {
            n165 = case shown="False" "HP 1" {
              tunnel: [0.0 ("Voltage") w445] -> w441
              frame #0 {
              }
              frame #1 {
                n166 = call "HP-ReadVoltagev2.vi"("String"="meas:volt:dc? 200,0.001", "HP-Mulitmeter\nGPIB Address"="GPIB HP") -> ("Voltage"=w445:dbl)  [unwired: 9 in]
              }
            }
          }
          frame #5 {
            n167 = case shown="True" "AH" {
              tunnel: [w450 w452] -> w447
              tunnel: [w450 w451] -> w448
              frame #0 {
                w450 = 0.0 ("Voltage")
              }
              frame #1 {
                n168 = call "AHRead2.vi"() -> ("loss"=w452:dbl, "capacitance"=w451:dbl)  [unwired: 8 in, 2 out]
              }
            }
          }
          frame #6 {
            n169 = Get Date/Time In Seconds() -> (seconds since 1Jan1904=w454:timestamp)
            n170 = To Double Precision Float(number=w454) -> (double precision float=w453:dbl)
          }
        }
        n171 = local read "Ramping Control"() -> (w372:u16)
        n172 = Build Array(w387, w386, w385, w384, w381, w380, w378, w379, w377, w376, w375, w369, w368, w370) -> (w374:dbl[])
        n173 = Array To Spreadsheet String(array=w374, 3:"%.8f" ("format string")) -> (spreadsheet string=w383:string)  [unwired: 1 in]
        n174 = Equal?(x=w372, y=w373) -> (x = y?=w371:bool)
        n175 = case shown="False" w371 {
          tunnel: w389 -> [w398 w399]
          tunnel: [w397 w399] -> w388
          tunnel: w383 -> [w396 _]
          frame #0 {
            n176 = local read "Messfile Refnum"() -> (w390:refnum<file>)
            n177 = Set File Position(refnum=w390, from (0:start)=1, error in=w398) -> (refnum out=w392:refnum<file>, error out=w393:errorcluster)  [unwired: 1 in]
            n178 = Write to Text File(file (use dialog)=w392, text=w396, error in=w393) -> (refnum out=w395:refnum<file>, error out=w394:errorcluster)  [unwired: 1 in, 1 out]
            n179 = Flush File(refnum=w395, error in=w394) -> (error out=w397:errorcluster)  [unwired: 1 out]
          }
          frame #1 {
          }
        }
      }
      frame #3 {
        n180 = local read "measured data"() -> (w460:dbl[][])
        n181 = Insert Into Array(array=w460, new element=w459) -> (w458:dbl[][])  [unwired: 2 in]
        n182 = case shown="0, Default" w457 {
          tunnel: w458 -> [w476 w490]
          tunnel: "Y Axis" -> [w478 w489]
          tunnel: "X Axis" -> [w466 w488]
          frame #0 {
            n183 = Index Array(array=w476, index (col)=1 ("disabled index (col)")) -> (element=w471:dbl[])  [unwired: 1 in]
            n184 = Index Array(array=w476, index (col)=0 ("disabled index (col)")) -> (element=w470:dbl[])  [unwired: 1 in]
            n185 = Square(x=w471) -> (x^2=w473:dbl[])
            n186 = Square(x=w470) -> (x^2=w474:dbl[])
            n187 = Index Array(array=w476, index (col)=w478) -> (element=w465:dbl[])  [unwired: 1 in]
            n188 = Divide(x=w471, y=w470) -> (x/y=w462:dbl[])
            n189 = Add(x=w474, y=w473) -> (x+y=w472:dbl[])
            n190 = Inverse Tangent(1:w462) -> (0:w461:dbl[])
            n191 = Square Root(x=w472) -> (sqrt(x)=w463:dbl[])
            n192 = Divide(x=w461, y=3.141592653589793) -> (x/y=w468:dbl[])
            n193 = Multiply(x=w468, y=180) -> (x*y=w464:dbl[])
            n194 = case shown="\"B\", Default" w466 {
              tunnel: w465 -> [w481 w484]
              tunnel: w464 -> [_ w483]
              tunnel: w463 -> [w480 _]
              frame #0 {
                n195 = Bundle(w480, "measured data"=w481) -> (w479:cluster{dbl[], "measured data":dbl[]})  [unwired: 1 in]
                n196 = local write "XY Graph"(w479) -> ()
              }
              frame #1 {
                n197 = Bundle(w483, "measured data"=w484) -> (w482:cluster{dbl[], "measured data":dbl[]})  [unwired: 1 in]
                n198 = local write "XY Graph"(w482) -> ()
              }
            }
          }
          frame #1 {
            n199 = Index Array(array=w490, index (col)=w488) -> (element=w487:dbl[])  [unwired: 1 in]
            n200 = Index Array(array=w490, index (col)=w489) -> (element=w486:dbl[])  [unwired: 1 in]
            n201 = Bundle("measured data"=w487, "measured data"=w486) -> (w485:T2)  [unwired: 1 in]
            n202 = local write "XY Graph"(w485) -> ()
          }
        }
        n203 = local write "measured data"(w458) -> ()
      }
    }
    n204 = local read "Ramping Control"() -> (w256:u16)
    n205 = case shown="3" w256 {
      selector: w256 -> [w492 w507 w530 w534 w549]
      tunnel: w255 -> [_ w510 _ w537 w554]
      tunnel: w254 -> [_ w509 _ w536 w553]
      tunnel: [w491 w508 w529 w535 w552] -> w253
      tunnel: [w492 w507 w530 w534 w549] -> w251
      tunnel: w250 -> [_ _ _ w533 w551]
      tunnel: w249 -> [_ _ _ _ w548]
      tunnel: w248 -> [_ _ _ _ w547]
      tunnel: w247 -> [_ w499 _ _ _]
      tunnel: w246 -> [w491 w495 w529 w531 w546]
      frame #0 {
      }
      frame #1 {
        w502 = T9."HOLDING" ("y")
        n206 = local read "Number of lines"() -> (w496:i32)
        n207 = local read "Starting index"() -> (w498:i32)
        n208 = call <userlib>:"Get Ramping Mode.vi"("Communications Config"=w510, "error in"=w495) -> ("Ramping Mode"=w505:T10, "error out"=w506:T5)  [unwired: 1 out]
        n209 = call <userlib>:"Get Ramping Mode.vi"("Communications Config"=w509, "error in"=w506) -> ("Ramping Mode"=w504:T10, "error out"=w508:T5)  [unwired: 1 out]
        n210 = Less?(x=w498, y=w496) -> (x < y?=w497:bool)
        n211 = Equal?(x=w505, y=w502) -> (x = y?=w501:bool)
        n212 = Equal?(x=w504, y=w502) -> (x = y?=w500:bool)
        n213 = Compound Arithmetic op=AND(w501, w500) -> (w503:bool)
        n214 = case shown="True" w503 {
          tunnel: w499 -> [_ w514]
          tunnel: w497 -> [_ w513]
          tunnel: "Wait between \nVectors (ms)" -> [_ w512]
          tunnel: "Wait between \nVectors" -> [_ w511]
          frame #0 {
          }
          frame #1 {
            n215 = case shown="1" w514 {
              tunnel: w513 -> [_ w519]
              tunnel: w512 -> [_ w518]
              tunnel: w511 -> [_ w517]
              frame #0 {
                w516 = u16 2 items=["NEXT VECTOR", "RAMPING", "HOLDING", "PAUSE", "ZERO"] ("Ramping Control")
                n216 = local write "STATUS"("Holding at current vector. Set Ramping Mode to NEXT VECTOR to continue." ("STATUS")) -> ()
                n217 = local write "Ramping Control"(w516) -> ()
              }
              frame #1 {
                # "Go to NEXT VECTOR automatically"
                n218 = case shown="True" w519 {
                  tunnel: w518 -> [_ w523]
                  tunnel: w517 -> [_ w522]
                  frame #0 {
                    w521 = u16 2 items=["NEXT VECTOR", "RAMPING", "HOLDING", "PAUSE", "ZERO"] ("Ramping Control")
                    n219 = local write "STATUS"("Holding at current vector. Set Ramping Mode to NEXT VECTOR to continue." ("STATUS")) -> ()
                    n220 = local write "Ramping Control"(w521) -> ()
                  }
                  frame #1 {
                    n221 = stacked-sequence {
                      tunnel: w523 -> [w525 _]
                      tunnel: w522 -> [w524 _]
                      frame #0 {
                        n222 = case shown="True" w524 {
                          tunnel: w525 -> [_ w526]
                          frame #0 {
                          }
                          frame #1 {
                            n223 = Wait (ms)(milliseconds to wait=w526) -> ()  [unwired: 1 out]
                          }
                        }
                      }
                      frame #1 {
                        w528 = u16 0 items=["NEXT VECTOR", "RAMPING", "HOLDING", "PAUSE", "ZERO"] ("Ramping Control")
                        n224 = local write "Ramping Control"(w528) -> ()
                        n225 = local write "STATUS"("Go to NEXT VECTOR" ("STATUS")) -> ()
                      }
                    }
                  }
                }
              }
            }
          }
        }
      }
      frame #2 {
      }
      frame #3 {
        n226 = Not Equal?(x=w534, y=w533) -> (x != y?=w532:bool)
        n227 = case shown="False" w532 {
          tunnel: w537 -> [_ w545]
          tunnel: w536 -> [_ w544]
          tunnel: [w538 w542] -> w535
          tunnel: w531 -> [w538 w539]
          frame #0 {
          }
          frame #1 {
            w540 = u16 1 items=["RAMP", "PAUSE", "MANUAL UP", "MANUAL DOWN", "ZERO"] ("Ramping Mode")
            n228 = call <userlib>:"Set Ramping Mode.vi"("error in"=w539, "Ramping Mode"=w540, "Communications Config"=w545) -> ("error out"=w543:T5)
            n229 = call <userlib>:"Set Ramping Mode.vi"("error in"=w543, "Ramping Mode"=w540, "Communications Config"=w544) -> ("error out"=w542:T5)
            n230 = local write "STATUS"("All Programmers are PAUSED. Set Ramping Mode to NEXT VECTOR to continue." ("STATUS")) -> ()
          }
        }
      }
      frame #4 {
        n231 = Not Equal?(x=w549, y=w551) -> (x != y?=w550:bool)
        n232 = case shown="False" w550 {
          tunnel: w554 -> [_ w563]
          tunnel: w553 -> [_ w562]
          tunnel: [w555 w558] -> w552
          tunnel: w548 -> [_ w561]
          tunnel: w547 -> [_ w560]
          tunnel: w546 -> [w555 w556]
          frame #0 {
          }
          frame #1 {
            w557 = u16 4 items=["RAMP", "PAUSE", "MANUAL UP", "MANUAL DOWN", "ZERO"] ("Ramping Mode")
            n233 = local write "STATUS"("Zeroing vector." ("STATUS")) -> ()
            n234 = call <userlib>:"Set Ramping Mode.vi"("error in"=w556, "Ramping Mode"=w557, "Communications Config"=w563) -> ("error out"=w566:T5)
            n235 = call <userlib>:"Set Ramping Mode.vi"("error in"=w566, "Ramping Mode"=w557, "Communications Config"=w562) -> ("error out"=w559:T5)
            n236 = call <userlib>:"Set Current Ramp Rate.vi"("Communications Config"=w563, "Ramp Rate (A/sec)"=w561, "error in"=w559) -> ("error out"=w564:T5)  [unwired: 2 in]
            n237 = call <userlib>:"Set Current Ramp Rate.vi"("Communications Config"=w562, "Ramp Rate (A/sec)"=w560, "error in"=w564) -> ("error out"=w558:T5)  [unwired: 2 in]
          }
        }
      }
    }
    n238 = local read "Continue Execution?"() -> (w252:bool)
  }
  n239 = case shown="0, Default" w30 {
    tunnel: w26 -> [w569 _ _]
    tunnel: w24 -> [w568 w572 w573]
    tunnel: [w567 w571 w573] -> w31
    tunnel: w25 -> [_ w570 _]
    frame #0 {
      n240 = call <userlib>:"430_TCP_Close.vi"("error in (no error)"=w568, "connection ID"=w569) -> ("error out"=w567:errorcluster)  [unwired: 1 out]
    }
    frame #1 {
      n241 = call <userlib>:"430_RS232_Close.vi"("error in (no error)"=w572, "VISA resource name"=w570) -> ("error out"=w571:errorcluster)  [unwired: 1 in]
    }
    frame #2 {
    }
  }
  n242 = case shown="0, Default" w29 {
    tunnel: w28 -> [w576 _ _]
    tunnel: w31 -> [w575 w579 w580]
    tunnel: [w574 w578 w580] -> w21
    tunnel: w27 -> [_ w577 _]
    frame #0 {
      n243 = call <userlib>:"430_TCP_Close.vi"("error in (no error)"=w575, "connection ID"=w576) -> ("error out"=w574:errorcluster)  [unwired: 1 out]
    }
    frame #1 {
      n244 = call <userlib>:"430_RS232_Close.vi"("error in (no error)"=w579, "VISA resource name"=w577) -> ("error out"=w578:errorcluster)  [unwired: 1 in]
    }
    frame #2 {
    }
  }
  "error out" <- w21
  n245 = local read "Magnetic Field Units"() -> (w48:u16)
  n246 = local read "Coordinate System"() -> (w49:u16)
  n247 = while {
    tunnel: "Starting index" -> [w588]
    tunnel: w23 -> [w594]
    tunnel: w22 -> [w595]
    tunnel: w48 -> [w596]
    tunnel: w49 -> [w597]
    tunnel: w46 -> [w600]
    tunnel: "Max Ramp Rate - Y Axis (A/s)" -> [w584]
    tunnel: "Max Ramp Rate - Z Axis (A/s)" -> [w583]
    tunnel: "Magnitude Limit (kG)" -> [w585]
    tunnel: "User defined Ramp Rate (T/min)" -> [w582]
    tunnel: "User defined Ramp Rate (T/min)" -> [w581]
    i -> [w587]
    stop <- w589 continue-if-true
    n248 = local read "Field Values"() -> (w591:string[][])
    n249 = Add(x=w588, y=w587) -> (x+y=w586:i32)
    n250 = while "Wait for NEXT VECTOR setting by operator." {
      tunnel: [w604] -> w599
      tunnel: w600 -> [w604]
      stop <- w605 continue-if-true
      w603 = u16 0 items=["NEXT VECTOR", "RAMPING", "HOLDING", "PAUSE", "ZERO"] ("Ramping Control")
      n251 = local read "Ramping Control"() -> (w606:u16)
      n252 = Not Equal?(x=w603, y=w606) -> (x != y?=w605:bool)
    }
    n253 = stacked-sequence {
      tunnel: w586 -> [w608 _ w614 _]
      frame #0 {
        (unwired) -2
        n254 = Subtract(x=w608, y=2) -> (x-y=w611:i32)
        n255 = Bundle(w611, -2) -> (w609:cluster{i32, i32})  [unwired: 1 in]
        n256 = property on="Field Values" class="Tbl (strict)"("Active Cell:Active Cell"=w609) -> ()  [unwired: 2 in, 2 out]
      }
      frame #1 {
        n257 = local read "Normal color"() -> (w612:u32)
        n258 = property on="Field Values" class="Tbl (strict)"("Active Cell:Cell Background Color"=w612) -> ()  [unwired: 2 in, 2 out]
      }
      frame #2 {
        n259 = Decrement(x=w614) -> (x-1=w613:i32)
        n260 = Bundle(w613, -2) -> (w616:cluster{i32, i32})  [unwired: 1 in]
        n261 = property on="Field Values" class="Tbl (strict)"("Active Cell:Active Cell"=w616) -> ()  [unwired: 2 in, 2 out]
      }
      frame #3 {
        n262 = property on="Field Values" class="Tbl (strict)"("Active Cell:Cell Background Color"="Highlight color") -> ()  [unwired: 2 in, 2 out]
      }
    }
    n263 = Index Array(array=w591, index (row)=w586) -> (element=w598:string[])  [unwired: 1 in]
    n264 = local write "Starting index"(w586) -> ()
    n265 = Add(x=1, y=w586) -> (x+y=w601:i32)
    n266 = Number To Decimal String(number=w601) -> (decimal integer string=w590:string)  [unwired: 1 in]
    n267 = stacked-sequence {
      tunnel: [_ w642] -> w592
      tunnel: [_ w641] -> w593
      tunnel: w599 -> [_ w637]
      tunnel: w598 -> [_ w636]
      tunnel: w597 -> [_ w635]
      tunnel: w596 -> [_ w634]
      tunnel: w595 -> [_ w633]
      tunnel: w594 -> [_ w632]
      tunnel: w590 -> [_ w631]
      tunnel: w585 -> [_ w629]
      tunnel: w584 -> [_ w628]
      tunnel: w583 -> [_ w623]
      tunnel: w582 -> [_ w627]
      tunnel: w581 -> [_ w626]
      frame #0 {
        w621 = u16 1 items=["NEXT VECTOR", "RAMPING", "HOLDING", "PAUSE", "ZERO"] ("Ramping Control")
        n268 = local write "Ramping Control"(w621) -> ()
      }
      frame #1 {
        n269 = call <userlib>:"Set 2D Next Vector_entwurf.vi"("Coordinate System"=w635, "Magnetic Field Units"=w634, 3:"User defined Ramp Rate (T/min)"=w626, "Magnitude Limit (kG)"=w629, "Y-Axis Communications Config"=w633, "Input Vector"=w636, "Z-Axis Communications Config"=w632, 10:"User defined Ramp Rate (T/min)"=w627, "Max Ramp Rate - Y Axis (A/s)"=w628, "error in"=w637, "Max Ramp Rate - Z Axis (A/s)"=w623) -> ("Y-Axis Ramp Rate (T/min)"=→"Current Ramp Rate Y (T/min)":dbl, "Within Limits?"=w642:bool, "Ramp Rate along Vector (T/min)"=→"Ramp Rate along Vector (T/min)":dbl, "Z-Axis Ramp Rate (T/min)"=→"Current Ramp Rate Z (T/min)":dbl, "All Instruments Responded?"=w641:bool, "error out"=w630:T5)  [unwired: 3 in]
        n270 = Concatenate Strings("Ramping to field vector " ("STATUS"), w631, "..." ("STATUS")) -> (w638:string)
        n271 = local write "error in"(w630) -> ()
        n272 = local write "STATUS"(w638) -> ()
      }
    }
    n273 = case shown="True" w592 {
      tunnel: w593 -> [_ w619]
      frame #0 {
        n274 = local write "STATUS"("Vector magnitude limt or maximum coil current exceeded. Vector ignored. VI halted." ("STATUS")) -> ()
      }
      frame #1 {
        n275 = case shown="True" w619 {
          frame #0 {
            n276 = local write "STATUS"("Not all programmers responded. VI halted." ("STATUS")) -> ()
          }
          frame #1 {
          }
        }
      }
    }
    n277 = Compound Arithmetic op=AND(w593, w592) -> (w589:bool)
    n278 = local write "Continue Execution?"(w589) -> ()
  }
